vi "Klinger GetAxisParams.vi"(0 "Axe":u8(ring) items=["W", "X", "Y", "Z"], 11 "error in":errorcluster) -> (3 "TypeMouv":i32(ring) caption="Type de mouvement" items=["Linéaire", "Rotation"], 4 "Nom de l'axe":string, 6 "Type":i32(ring) caption="Type de moteur" items=["UE30", "UE72"], 8 "FactConv":dbl=0.01 caption="Facteur de\nConversion\n(m/pas ou °/pas)", 10 "CorrParams":T1={"CorrActive"=FALSE, "ErreurLim"=0.1, "NbrEssais"=3} caption="Paramètres de correction de position" {"NbrEssais" min=1 max=5 step=1; "ErreurLim" min=0.0 max=10.0 step=0.1 format="%#.1f"}, 13 "Encodeur":bool caption="Possède un\nEncodeur", 14 "MiseàZéro":bool caption="Possède un\nInterrupteur d'origine", 15 "error out":errorcluster)   [LabVIEW 2010]
doc: "Ce Vi lit les paramètres des différents axes moteur, qui sont enregistrer dans un fichier .ini."
uses:
  <vilib>/Utility/config.llb/Read Key (I32).vi
  <vilib>/Utility/config.llb/Read Key (Boolean).vi
  <vilib>/Utility/config.llb/Read Key (Double).vi
  <vilib>/Utility/config.llb/Read Key (String).vi
  <vilib>/Utility/config.llb/NI_LVConfig.lvlib
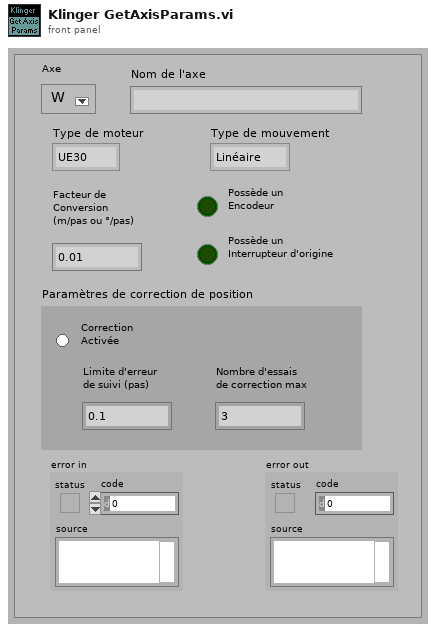
[diagram p1: front panel]
types:
  T1 = cluster{"CorrActive":bool, "ErreurLim":dbl, "NbrEssais":i32}
  T2 = typedef "NI_LVConfig.lvlib/Config Data RefNum.ctl" = refnum<k1>
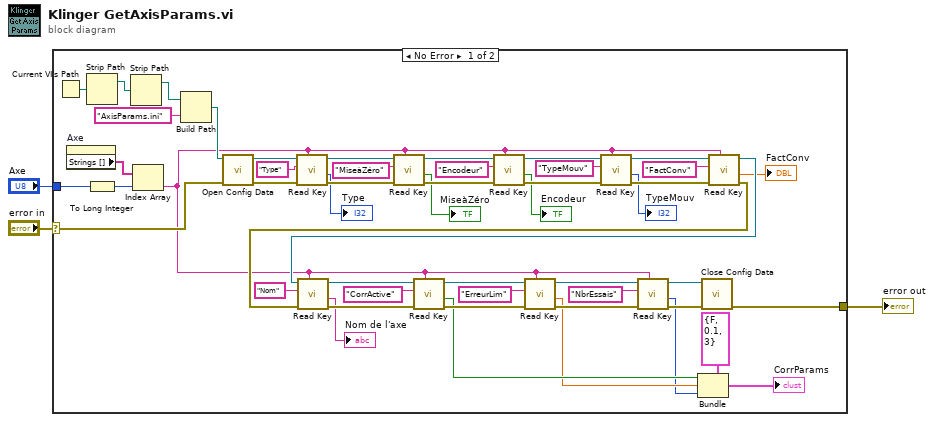
[diagram p0: block diagram]
diagram:
  n1 = case shown="No Error" "error in" {
    selector: "error in" -> [w49 w55]
    tunnel: "Axe" -> [w48 _]
    tunnel: [w16 w55] -> w2
    frame No Error {
      n2 = Current VI's Path() -> (path=w54:path)
      n3 = property on="Axe" class="Ring (strict)"() -> ("Strings []"=w46:string[])  [unwired: 2 in, 2 out]
      n4 = Strip Path(path=w54) -> (stripped path=w53:path)  [unwired: 1 out]
      n5 = To Long Integer(number=w48) -> (32bit integer=w47:i32)
      n6 = Strip Path(path=w53) -> (stripped path=w52:path)  [unwired: 1 out]
      n7 = Index Array(array=w46, index=w47) -> (element=w15:string)
      n8 = Build Path(base path=w52, name or relative path="AxisParams.ini") -> (appended path=w50:path)
      n9 = call <vilib>:"Open Config Data.vi"("error in (no error)"=w49, "configuration file path"=w50) -> ("error out"=w36:errorcluster, "refnum"=w37:T2)  [unwired: 7 in, 1 out]
      n10 = call-poly <vilib>:"Read Key.vi"("section"=w15, "error in (no error)"=w36, "key"="Type", "refnum"=w37) -> ("error out"=w33:errorcluster, "value"=→"Type":i32, "refnum out"=w35:T2)  [unwired: 4 in, 1 out]
      n11 = call-poly <vilib>:"Read Key.vi"("section"=w15, "error in (no error)"=w33, "key"="MiseàZéro", "refnum"=w35) -> ("error out"=w32:errorcluster, "value"=→"MiseàZéro":bool, "refnum out"=w27:T2)  [unwired: 4 in, 1 out]
      n12 = call-poly <vilib>:"Read Key.vi"("section"=w15, "error in (no error)"=w32, "key"="Encodeur", "refnum"=w27) -> ("error out"=w31:errorcluster, "value"=→"Encodeur":bool, "refnum out"=w28:T2)  [unwired: 4 in, 1 out]
      n13 = call-poly <vilib>:"Read Key.vi"("section"=w15, "error in (no error)"=w31, "key"="TypeMouv", "refnum"=w28) -> ("error out"=w30:errorcluster, "value"=→"TypeMouv":i32, "refnum out"=w29:T2)  [unwired: 4 in, 1 out]
      n14 = call-poly <vilib>:"Read Key.vi"("section"=w15, "error in (no error)"=w30, "key"="FactConv", "refnum"=w29) -> ("error out"=w25:errorcluster, "value"=→"FactConv":dbl, "refnum out"=w26:T2)  [unwired: 4 in, 1 out]
      n15 = call-poly <vilib>:"Read Key.vi"("section"=w15, "error in (no error)"=w25, "key"="Nom", "refnum"=w26) -> ("error out"=w23:errorcluster, "value"=→"Nom de l'axe":string, "refnum out"=w24:T2)  [unwired: 4 in, 1 out]
      n16 = call-poly <vilib>:"Read Key.vi"("section"=w15, "error in (no error)"=w23, "key"="CorrActive", "refnum"=w24) -> ("error out"=w21:errorcluster, "value"=w7:bool, "refnum out"=w22:T2)  [unwired: 4 in, 1 out]
      n17 = call-poly <vilib>:"Read Key.vi"("section"=w15, "error in (no error)"=w21, "key"="ErreurLim", "refnum"=w22) -> ("error out"=w19:errorcluster, "value"=w6:dbl, "refnum out"=w20:T2)  [unwired: 4 in, 1 out]
      n18 = call-poly <vilib>:"Read Key.vi"("section"=w15, "error in (no error)"=w19, "key"="NbrEssais", "refnum"=w20) -> ("error out"=w17:errorcluster, "value"=w5:i32, "refnum out"=w18:T2)  [unwired: 4 in, 1 out]
      n19 = Bundle(cluster=T1 {"CorrActive"=FALSE, "ErreurLim"=0.1, "NbrEssais"=3} ("CorrParams"), "CorrActive"=w7, "ErreurLim"=w6, "NbrEssais"=w5) -> (→"CorrParams":T1)
      n20 = call <vilib>:"Close Config Data.vi"("error in (no error)"=w17, "refnum"=w18) -> ("error out"=w16:errorcluster)  [unwired: 8 in, 1 out]
    }
    frame Error {
    }
  }
  "error out" <- w2
